vi "Add items.vi"(9 "Value":refnum<class "IMessagePackObject.lvclass">, 10 "Key":refnum<class "IMessagePackObject.lvclass">, 11 "MsgPackMap in":refnum<class "MsgPackMap.lvclass">) -> (3 "MsgPackMap out":refnum<class "MsgPackMap.lvclass">)   [LabVIEW 2020, in "MessagePack.lvlib" / "MsgPackMap.lvclass"]
uses:
  MsgPackMap.lvclass
  MsgPackMap.lvclass/MsgPackMap.ctl
  IMessagePackObject/IMessagePackObject.lvclass
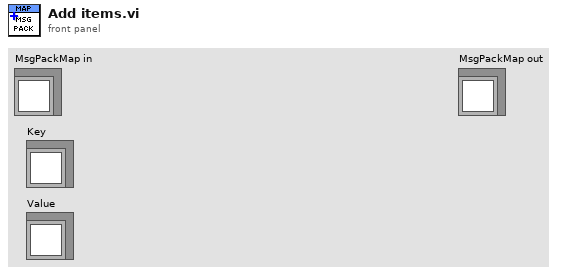
[diagram p1: front panel]
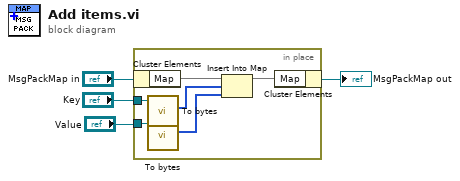
[diagram p0: block diagram]
diagram:
  n1 = in-place {
    in-place-border: "Key" -> [w8]
    in-place-border: "Value" -> [w7]
    n2 = in-place-cluster #1("MsgPackMap in") -> ("Map"=w10:map{u8[], u8[]})
    n3 = call-dynamic "To bytes.vi"("IMessagePackObject in"=w8) -> ("Array"=w6:u8[])  [unwired: 9 in, 1 out]
    n4 = call-dynamic "To bytes.vi"("IMessagePackObject in"=w7) -> ("Array"=w5:u8[])  [unwired: 9 in, 1 out]
    n5 = Insert Into Map(map in=w10, key=w6, value=w5) -> (map out=w9:map{u8[], u8[]})  [unwired: 2 out]
    n6 = in-place-cluster #1("Map"=w9) -> (→"MsgPackMap out":refnum<class "MsgPackMap.lvclass">)
  }
